vi "start sr400.vi"(11 "GPIB Address":string) -> ()   [LabVIEW 2011]
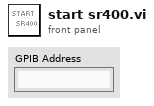
[diagram p1: front panel]
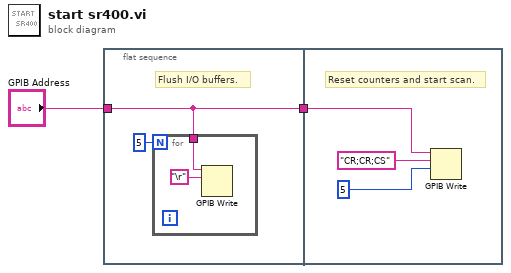
[diagram p0: block diagram]
diagram:
  n1 = flat-sequence {
    tunnel: "GPIB Address" -> [w3]
    tunnel: [w3] -> w2
    tunnel: w2 -> [w9]
    frame #0 {
      # "Flush I/O buffers."
      n2 = for {
        N: 5 -> [_]
        tunnel: w3 -> [w5]
        n3 = GPIB Write(0:w5, 1:"\r") -> ()  [unwired: 3 in, 2 out]
      }
    }
    frame #1 {
      # "Reset counters and start scan."
      n4 = GPIB Write(0:w9, 1:"CR;CR;CS", 2:i16 5 ("mode (0)")) -> ()  [unwired: 2 in, 2 out]
    }
  }
